vi "Set Window Title.vi"(8 "error in (no error)":errorcluster, 10 "FP Window:Title":string, 11 "Station in":refnum<class "Station.lvclass">) -> (0 "error out":errorcluster, 3 "Station out":refnum<class "Station.lvclass">)   [LabVIEW 2021, in "Station.lvlib" / "Station.lvclass"]
uses:
  Station.lvclass
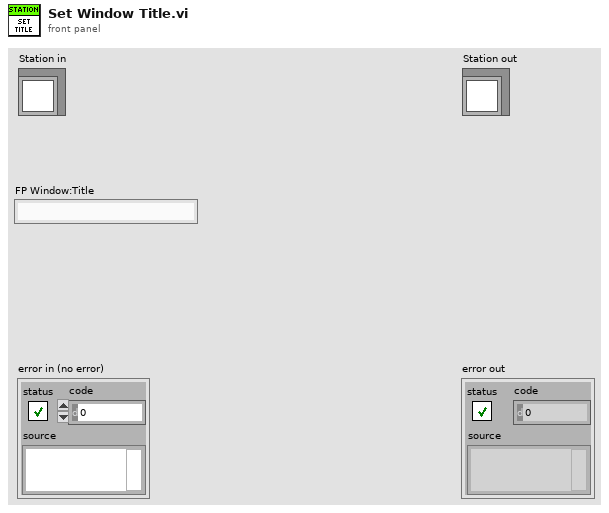
[diagram p1: front panel]
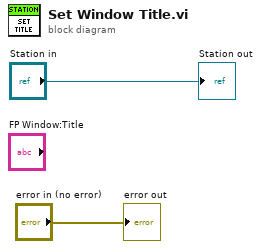
[diagram p0: block diagram]
diagram:
  "error out" <- "error in (no error)"
  "Station out" <- "Station in"
